vi "1B_Find Offset.vi"(0 "Waveform":waveform(dbl), 1 "Smoothing Strength":T2=enum."10", 2 "Offset Calculation Method":T1=enum."Precise") -> (3 "Offset":dbl=3.799820325600689 format="%0.2f")   [LabVIEW 2010]
uses:
  FilterStrength.ctl
  1B_Offset Calculation Method.ctl
  <vilib>/Analysis/NI_AALBase.lvlib
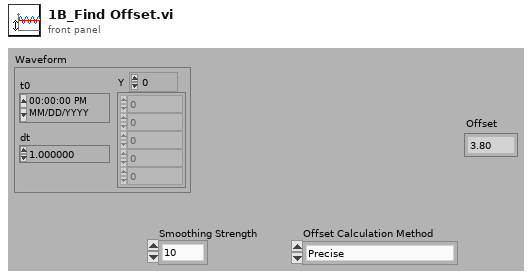
[diagram p1: front panel]
types:
  T1 = typedef "1B_Offset Calculation Method.ctl" = enum16{"Obsolete", "Precise", "Simple"}
  T2 = typedef "FilterStrength.ctl" = enum16{"Off", "10", "20", "50", "100", "200", "500", "1000"}
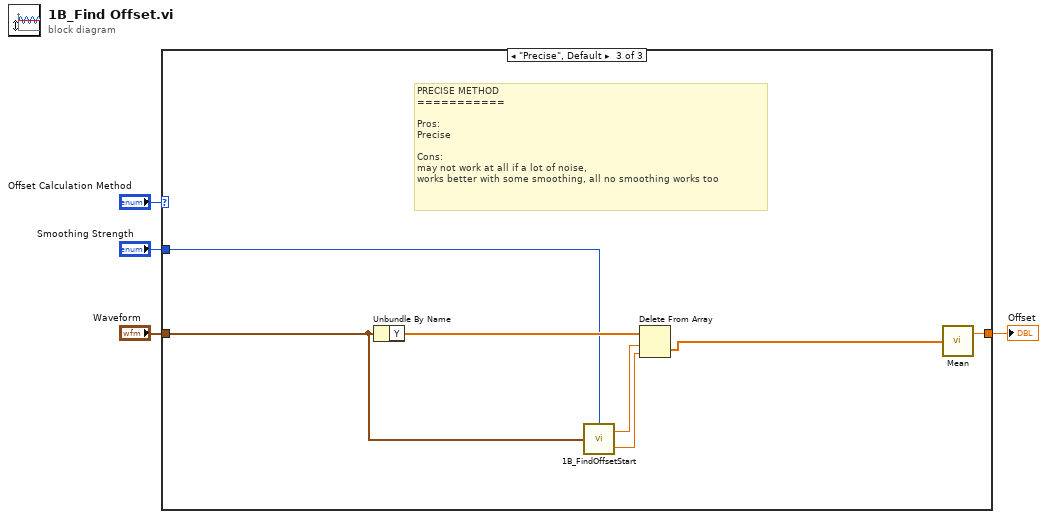
[diagram p0: block diagram]
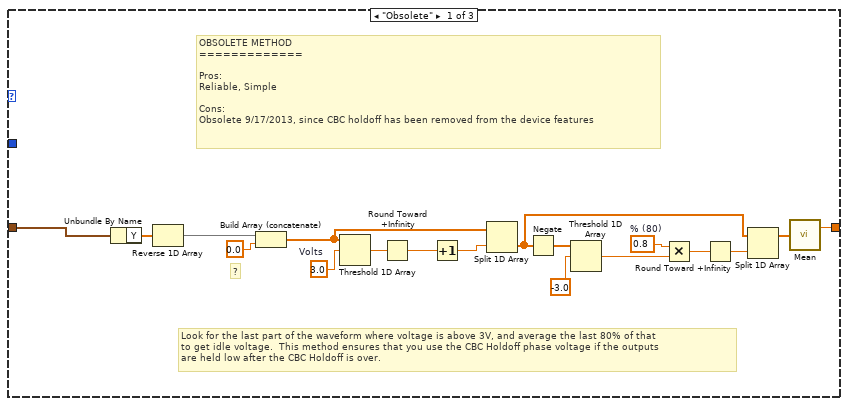
[diagram p2: hidden frame]
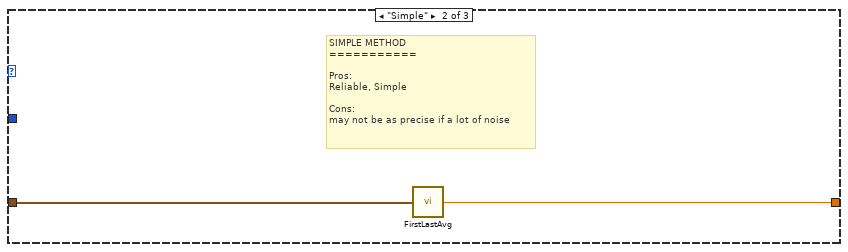
[diagram p3: hidden frame]
diagram:
  n1 = case shown="\"Precise\", Default" "Offset Calculation Method" {
    tunnel: [w5 w24 w25] -> w3
    tunnel: "Waveform" -> [w6 w23 w26]
    tunnel: "Smoothing Strength" -> [_ _ w27]
    frame "Obsolete" {
      w14 = 0.8  # % (80)
      w9 = 3.0  # Volts
      # "OBSOLETE METHOD\n=============\n\nPros:\nReliable, Simple\n\nCons:\nObsolete 9/17/2013, since CBC holdoff has been removed from the device features"
      # "?"
      # "Look for the last part of the waveform where voltage is above 3V, and average the last 80% of that\nto get idle voltage.  This method ensures that you use the CBC Holdoff phase voltage if the outputs\nare held low after the CBC Holdoff is over."
      n2 = Unbundle By Name(w6) -> ("Y"=w19:dbl[])
      n3 = Reverse 1D Array(array=w19) -> (reversed array=w7:dbl[])
      n4 = Build Array (concatenate)(w7, 0.0 ("y")) -> (w20:dbl[])
      n5 = Threshold 1D Array(2:w9, 3:w20) -> (0:w10:dbl)  [unwired: 1 in]
      n6 = Round Toward +Infinity(x=w10) -> (ceil(x): smallest int >= x=w11:dbl)
      n7 = Increment(x=w11) -> (x+1=w17:dbl)
      n8 = Split 1D Array(array=w20, index=w17) -> (second subarray=w18:dbl[])  [unwired: 1 out]
      n9 = Negate(x=w18) -> (-x=w21:dbl[])
      n10 = Threshold 1D Array(2:-3.0 ("y"), 3:w21) -> (0:w13:dbl)  [unwired: 1 in]
      n11 = Multiply(x=w14, y=w13) -> (x*y=w15:dbl)
      n12 = Round Toward +Infinity(x=w15) -> (ceil(x): smallest int >= x=w16:dbl)
      n13 = Split 1D Array(array=w18, index=w16) -> (first subarray=w22:dbl[])  [unwired: 1 out]
      n14 = call <vilib>:"Mean.vi"("X"=w22) -> ("mean"=w5:dbl)  [unwired: 1 out]
    }
    frame "Simple" {
      # "SIMPLE METHOD\n===========\n\nPros:\nReliable, Simple\n\nCons:\nmay not be as precise if a lot of noise"
      n15 = call "FirstLastAvg.vi"("waveform"=w23) -> ("avg value"=w24:dbl)
    }
    frame "Precise", Default {
      # "PRECISE METHOD\n===========\n\nPros:\nPrecise\n\nCons:\nmay not work at all if a lot of noise,\nworks better with some smoothing, all no smoothing works too"
      n16 = Unbundle By Name(w26) -> ("Y"=w30:dbl[])
      n17 = call "1B_FindOffsetStart.vi"("waveform"=w26, "Smoothing Strength"=w27) -> ("floor Length"=w29:dbl, "start of floor index"=w28:dbl)
      n18 = Delete From Array(array=w30, length=w29, index=w28) -> (deleted portion=w31:dbl[])  [unwired: 1 out]
      n19 = call <vilib>:"Mean.vi"("X"=w31) -> ("mean"=w25:dbl)  [unwired: 1 out]
    }
  }
  "Offset" <- w3
